vi "任意波形脚本.vi"(8 "4-wire":bool, 11 "波形":waveform(dbl)) -> (3 "Script":string)   [LabVIEW 2020, in "功能选择.xctl"]
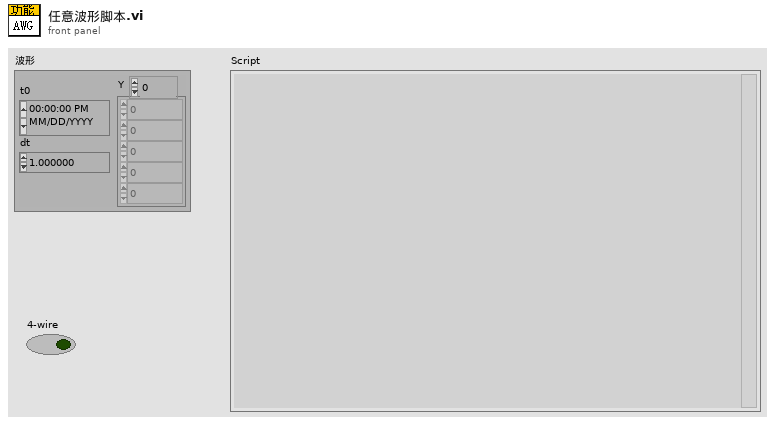
[diagram p1: front panel]
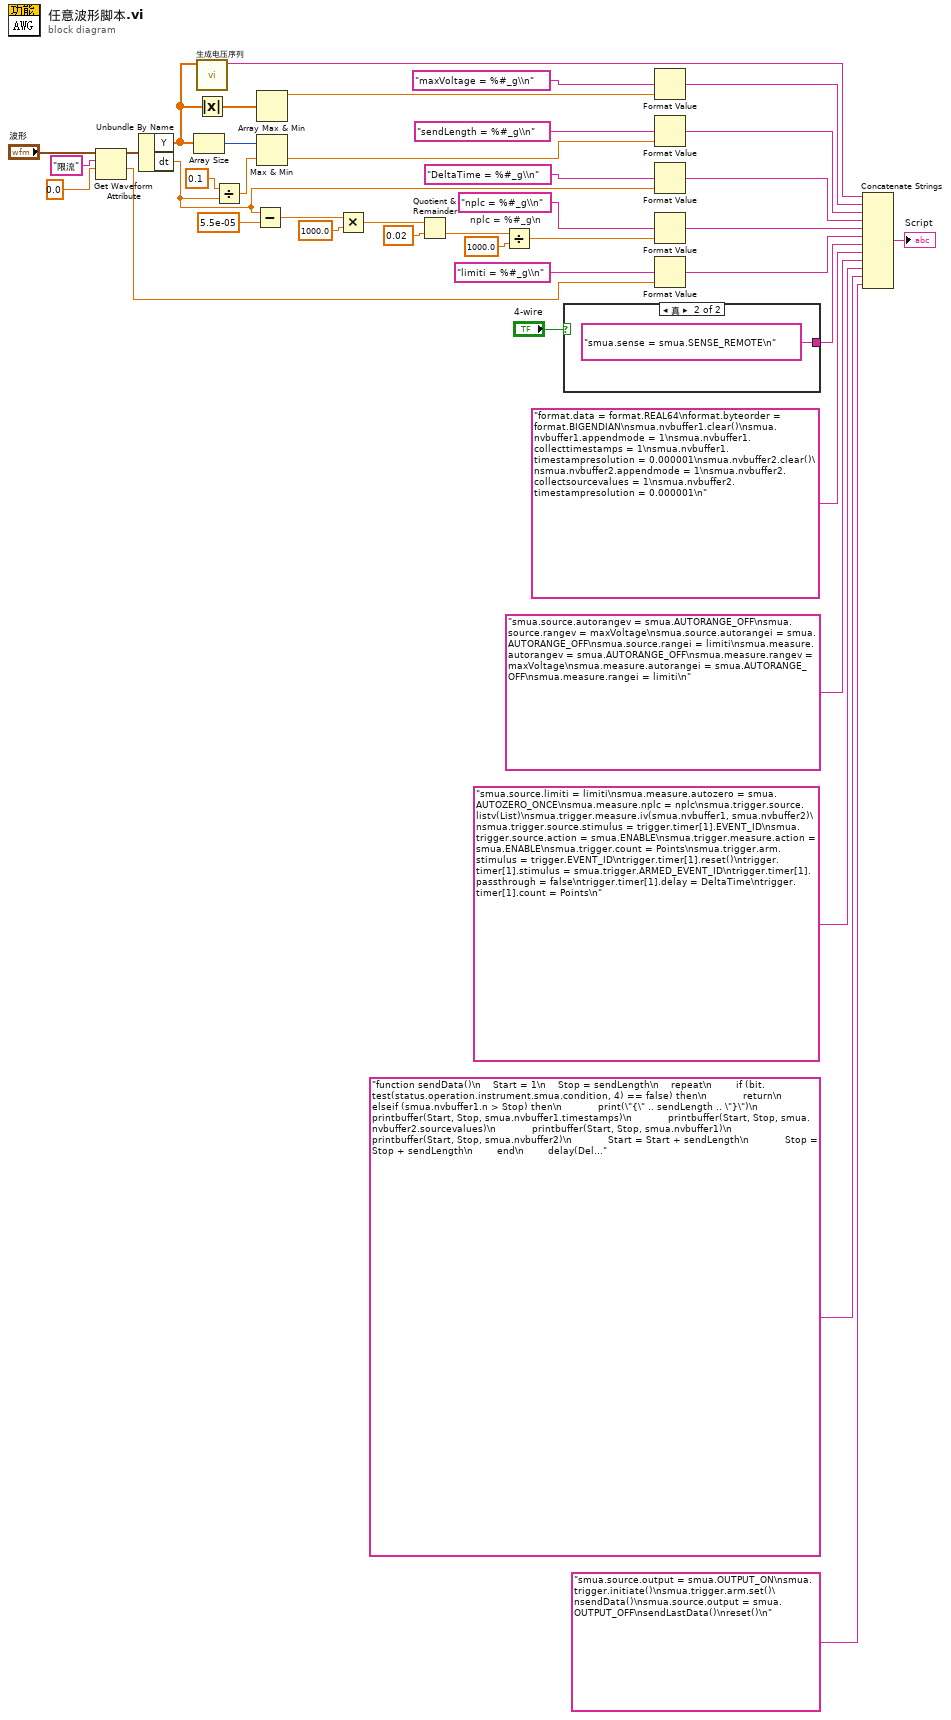
[diagram p0: block diagram]
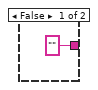
[diagram p2: hidden frame]
diagram:
  w32 = "nplc = %#_g\\n"  # nplc = %#_g\n
  n1 = Get Waveform Attribute(5:0.0, 6:"限流" ("名称"), 7:"波形") -> (1:w3:dbl, 3:w4:waveform(dbl))  [unwired: 1 in, 2 out]
  n2 = Unbundle By Name(w4) -> ("Y"=w14:dbl[], "dt"=w15:dbl)
  n3 = Array Size(array=w14) -> (size(s)=w13:i32)
  n4 = call "生成电压序列.vi"("电压序列"=w14) -> ("List"=w33:string)  [unwired: 10 in]
  n5 = Absolute Value(x=w14) -> (abs(x)=w35:dbl[])
  n6 = Divide(x=0.1, y=w15) -> (x/y=w12:dbl)
  n7 = Subtract(x=w15, y=5.5e-05) -> (x-y=w25:dbl)
  n8 = Array Max & Min(array=w35) -> (max value=w34:dbl)  [unwired: 3 out]
  n9 = Max & Min(x=w13, y=w12) -> (min(x,y)=w11:dbl)  [unwired: 1 out]
  n10 = Multiply(x=w25, y=1000.0) -> (x*y=w24:dbl)
  n11 = Quotient & Remainder(x=w24, y=0.02 ("x")) -> (floor(x/y)=w28:dbl)  [unwired: 1 out]
  n12 = Divide(x=w28, y=1000.0) -> (x/y=w21:dbl)
  n13 = case shown="真" "4-wire" {
    tunnel: ["" "smua.sense = smua.SENSE_REMOTE\n"] -> w2
    frame False {
    }
    frame True {
    }
  }
  n14 = Format Value(format string="maxVoltage = %#_g\\n" ("格式字符串"), value (0)=w34) -> (output string=w40:string)  [unwired: 1 in]
  n15 = Format Value(format string="sendLength = %#_g\\n" ("格式字符串"), value (0)=w11) -> (output string=w9:string)  [unwired: 1 in]
  n16 = Format Value(format string="DeltaTime = %#_g\\n" ("格式字符串"), value (0)=w15) -> (output string=w38:string)  [unwired: 1 in]
  n17 = Format Value(format string=w32, value (0)=w21) -> (output string=w36:string)  [unwired: 1 in]
  n18 = Format Value(format string="limiti = %#_g\\n" ("格式字符串"), value (0)=w3) -> (output string=w8:string)  [unwired: 1 in]
  n19 = Concatenate Strings(w33, w40, w9, w38, w36, w8, w2, "format.data = format.REAL64\nformat.byteorder = format.BIGENDIAN\nsmua.nvbuffer1.clear()\nsmua.nvbuffer1.appendmode = 1\nsmua.nvbuffer1.collecttimestamps = 1\nsmua.nvbuffer1.timestampresolution = 0.000001\nsmua.nvbuffer2.clear()\nsmua.nvbuffer2.appendmode = 1\nsmua.nvbuffer2.collectsourcevalues = 1\nsmua.nvbuffer2.timestampresolution = 0.000001\n", "smua.source.autorangev = smua.AUTORANGE_OFF\nsmua.source.rangev = maxVoltage\nsmua.source.autorangei = smua.AUTORANGE_OFF\nsmua.source.rangei = limiti\nsmua.measure.autorangev = smua.AUTORANGE_OFF\nsmua.measure.rangev = maxVoltage\nsmua.measure.autorangei = smua.AUTORANGE_OFF\nsmua.measure.rangei = limiti\n", "smua.source.limiti = limiti\nsmua.measure.autozero = smua.AUTOZERO_ONCE\nsmua.measure.nplc = nplc\nsmua.trigger.source.listv(List)\nsmua.trigger.measure.iv(smua.nvbuffer1, smua.nvbuffer2)\nsmua.trigger.source.stimulus = trigger.timer[1].EVENT_ID\nsmua.trigger.source.action = smua.ENABLE\nsmua.trigger.measure.action = smua.ENABLE\nsmua.trigger.count = Points\nsmua.trigger.arm.stimulus = trigger.EVENT_ID\ntrigger.timer[1].reset()\ntrigger.timer[1].stimulus = smua.trigger.ARMED_EVENT_ID\ntrigger.timer[1].passthrough = false\ntrigger.timer[1].delay = DeltaTime\ntrigger.timer[1].count = Points\n", "function sendData()\n    Start = 1\n    Stop = sendLength\n    repeat\n        if (bit.test(status.operation.instrument.smua.condition, 4) == false) then\n            return\n        elseif (smua.nvbuffer1.n > Stop) then\n            print(\"{\" .. sendLength .. \"}\")\n            printbuffer(Start, Stop, smua.nvbuffer1.timestamps)\n            printbuffer(Start, Stop, smua.nvbuffer2.sourcevalues)\n            printbuffer(Start, Stop, smua.nvbuffer1)\n            printbuffer(Start, Stop, smua.nvbuffer2)\n            Start = Start + sendLength\n            Stop = Stop + sendLength\n        end\n        delay(DeltaTime)\n    until (false)\nend\nfunction sendLastData()\n    Stop = smua.nvbuffer1.n\n    print(\"{\" .. Stop - Start + 1 .. \"}\")\n    printbuffer(Start, Stop, smua.nvbuffer1.timestamps)\n    printbuffer(Start, Stop, smua.nvbuffer2.sourcevalues)\n    printbuffer(Start, Stop, smua.nvbuffer1)\n    printbuffer(Start, Stop, smua.nvbuffer2)\n    print(\"{done}\")\nend\n", "smua.source.output = smua.OUTPUT_ON\nsmua.trigger.initiate()\nsmua.trigger.arm.set()\nsendData()\nsmua.source.output = smua.OUTPUT_OFF\nsendLastData()\nreset()\n") -> (→"Script":string)
